vi "DUAL GAUGE-Offset display.vi"(7 "W/R":bool, 8 "Fehler (Eingang)":errorcluster, 9 "Sensor 2 Set":dbl format="%.3e", 10 "Sensor 1 Set":dbl format="%.3e", 11 "Referenz in":refnum<visa-resource-name>) -> (0 "Cluster (Ausgang)":errorcluster, 1 "Sensor2 Get":dbl format="%.3e", 2 "Sensor 1 Get":dbl format="%.3e", 3 "Referenz out":refnum<visa-resource-name>)   [LabVIEW 2010, in "Dual Gauge.lvlib"]
uses:
  Dual Gauge.lvlib
panel:
  # "mbar"
  # "mbar"
  # "mbar"
  # "mbar"
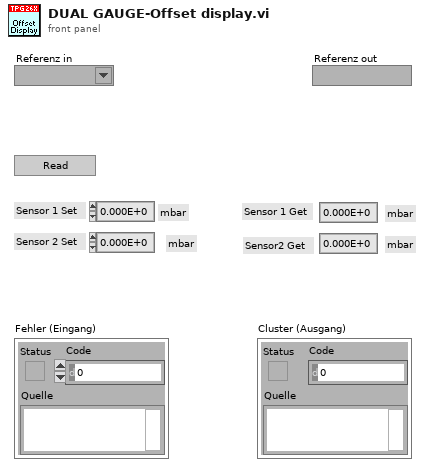
[diagram p1: front panel]
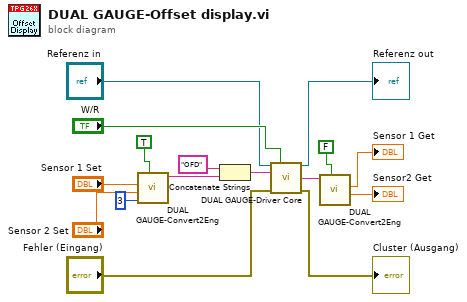
[diagram p0: block diagram]
diagram:
  n1 = call "DUAL GAUGE-Convert2Eng.vi"("W/R [W: Int in; Str out ]"=TRUE, "Kommastellen"=u8 3, "Eng2 in"="Sensor 2 Set", "Eng1 in"="Sensor 1 Set") -> ("String out"=w9:string)  [unwired: 5 in, 2 out]
  n2 = Concatenate Strings("OFD" ("Command"), w9) -> (w5:string)
  n3 = call "DUAL GAUGE-Driver Core.vi"("Referenz in"="Referenz in", "Write/Read"="W/R", "Command"=w5, "Fehler (Eingang)"="Fehler (Eingang)") -> ("Referenz out"=→"Referenz out":refnum<visa-resource-name>, "String Out"=w7:string, "Cluster (Ausgang)"=→"Cluster (Ausgang)":errorcluster)  [unwired: 9 in]
  n4 = call "DUAL GAUGE-Convert2Eng.vi"("W/R [W: Int in; Str out ]"=FALSE, "String in"=w7) -> ("Eng2 out"=→"Sensor2 Get":dbl, "Eng1 out"=→"Sensor 1 Get":dbl)  [unwired: 7 in, 1 out]
